vi "GET_Picture.vi"(8 "error in (no error)":errorcluster, 11 "Ants.lvclass in":refnum<class "Ants.lvclass">) -> (0 "error out":errorcluster, 2 "Picture":refnum<vi>, 3 "Ants.lvclass out":refnum<class "Ants.lvclass">)   [LabVIEW 2020, in "Ants.lvclass"]
uses:
  Ants.lvclass
  Ants.lvclass/Ants.ctl
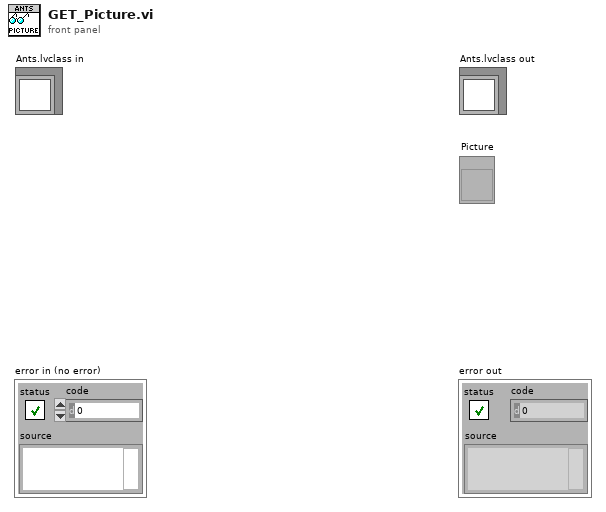
[diagram p1: front panel]
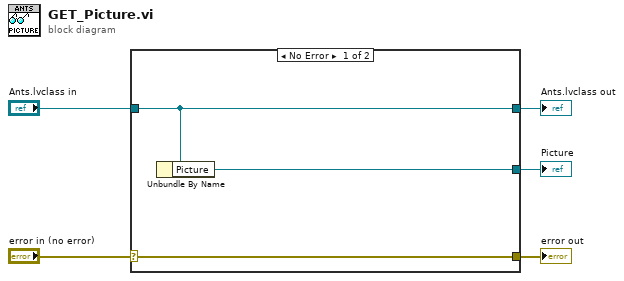
[diagram p0: block diagram]
diagram:
  n1 = case shown="No Error" "error in (no error)" {
    selector: "error in (no error)" -> [w8 w9]
    tunnel: [w8 w9] -> w4
    tunnel: [w7 w10] -> w2
    tunnel: "Ants.lvclass in" -> [w7 w10]
    tunnel: [w6 _] -> w1
    frame No Error {
      n2 = Unbundle By Name(w7) -> ("Picture"=w6:refnum<vi>)
    }
    frame Error {
    }
  }
  "error out" <- w4
  "Ants.lvclass out" <- w2
  "Picture" <- w1
